vi "检查曲线文件.vi"(8 "Error In":errorcluster, 11 "Folder Path":path caption="文件夹路径") -> (0 "Error Out":errorcluster, 1 "All Files in Dir":path[](array[path]) caption="目录中的所有文件", 2 "Exit?":bool, 3 "曲线文件路径":path)   [LabVIEW 2018]
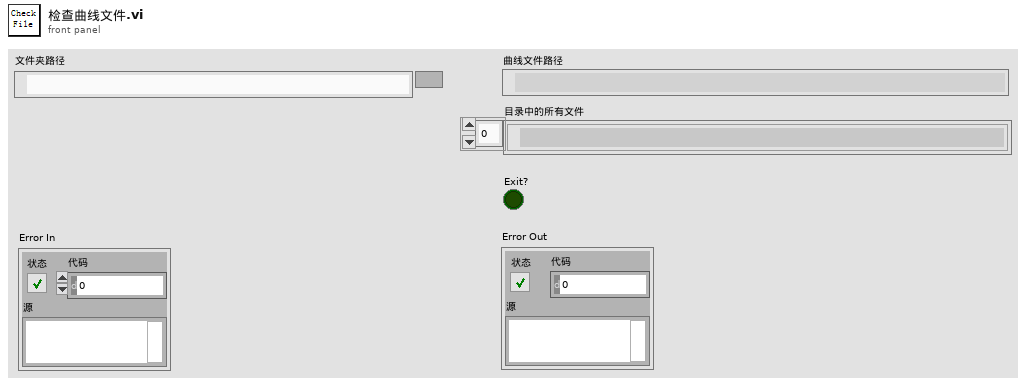
[diagram p1: front panel]
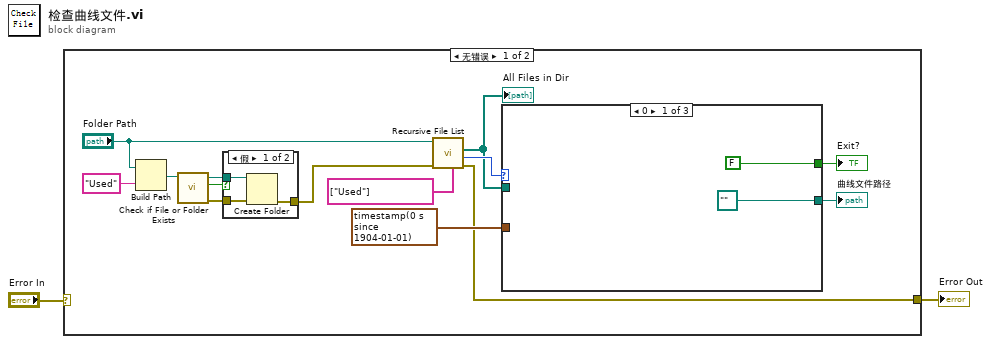
[diagram p0: block diagram]
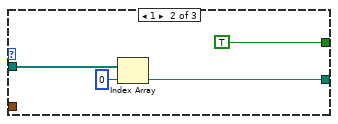
[diagram p3: hidden frame]
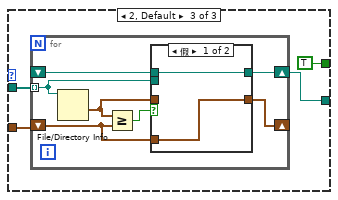
[diagram p4: hidden frame]
diagram:
  n1 = case shown="无错误" "Error In" {
    selector: "Error In" -> [_ w42]
    tunnel: [w10 w42] -> w1
    frame No Error {
      n2 = Build Path(base path="Folder Path", name or relative path="Used" ("名称或相对路径")) -> (appended path=w7:path)
      n3 = call <vilib>:"Check if File or Folder Exists.vi"("path"=w7) -> ("error out"=w4:errorcluster, "file or folder exists?"=w6:bool, "dup path"=w5:path)  [unwired: 8 in]
      n4 = case shown="假" w6 {
        tunnel: w5 -> [w19 _]
        tunnel: w4 -> [w18 w20]
        tunnel: [w17 w20] -> w3
        frame False {
          n5 = Create Folder(path (use dialog)=w19, error in=w18) -> (error out=w17:errorcluster)  [unwired: 1 in, 2 out]
        }
        frame True {
        }
      }
      n6 = call <vilib>:"Recursive File List.vi"("Folders to Exclude"=string[] ["Used"], "error in (no error)"=w3, "Folder Path"="Folder Path") -> ("error out"=w10:errorcluster, "Number of Files"=w15:i32, "All Files in Dir"=w14:path[])  [unwired: 4 in, 2 out]
      "All Files in Dir" <- w14
      n7 = case shown="0" w15 {
        tunnel: w14 -> [_ w26 w30]
        tunnel: [path "" w24 w28] -> w13
        tunnel: [FALSE TRUE TRUE] -> w12
        tunnel: timestamp(0 s since 1904-01-01) ("上次修改 2") -> [_ _ w29]
        frame 0 {
        }
        frame 1 {
          n8 = Index Array(array=w26, index=0 ("索引")) -> (element=w24:path)
        }
        frame 2, Default {
          n9 = for {
            tunnel: w30 -> [w34] mode=indexing
            shift-right: [w32] -> _
            shift-left: w29 -> [w31]
            shift-right: [w36] -> w28
            shift-left: _ -> [w35]
            n10 = File/Directory Info(path=w34) -> (last mod=w33:timestamp)  [unwired: 1 in, 6 out]
            n11 = Greater Or Equal?(x=w33, y=w31) -> (x >= y?=w37:bool)
            n12 = case shown="假" w37 {
              tunnel: w35 -> [w39 _]
              tunnel: [w39 w41] -> w36
              tunnel: w34 -> [_ w41]
              tunnel: w33 -> [_ w40]
              tunnel: [w38 w40] -> w32
              tunnel: w31 -> [w38 _]
              frame False {
              }
              frame True {
              }
            }
          }
        }
      }
      "曲线文件路径" <- w13
      "Exit?" <- w12
    }
    frame Error {
    }
  }
  "Error Out" <- w1
